vi "1D Rational Polynomial Evaluation.vi"   [LabVIEW 2017, in "NI_AALPro.lvlib"]
doc: "Evaluates a rational polynomial at the points you specify in <B>A</B>. <B>P(x)</B> and <B>Q(x)</B> specify the numerator and denominator polynomial coefficients, respectively. The data types you wire to the <B>P(x)</B> and <B>Q(x)</B> inputs determine the polymorphic instance to use."
uses:
  NI_AALPro.lvlib
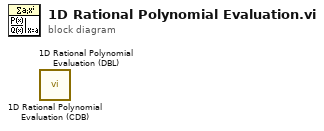
[diagram p0: block diagram]
diagram:
  n1 = call "1D Rational Polynomial Evaluation (CDB).vi"() -> ()  [unwired: 10 in, 2 out]
  n2 = call "1D Rational Polynomial Evaluation (DBL).vi"() -> ()  [unwired: 10 in, 2 out]
